vi "addBoolean[]Element.vi"(7 "Name":string, 8 "error in (no error)":errorcluster, 9 "Value":bool[](array[boolean]), 10 "Replace? (false)":bool, 11 "tBSONDocument in":refnum<class "tBSONDocument.lvclass">) -> (0 "error out":errorcluster, 3 "tBSONDocument out":refnum<class "tBSONDocument.lvclass">)   [LabVIEW 2013, in "BSON.lvlib" / "tBSONDocument.lvclass"]
doc: "Adds an array of booleans to a BSON document."
uses:
  tBSONDocument.lvclass
  BSONElements/tBSONBoolean/tBSONBoolean.lvclass
  tBSONElement/tBSONElement.lvclass
  BSONElements/tBSONBoolean/setValue.vi
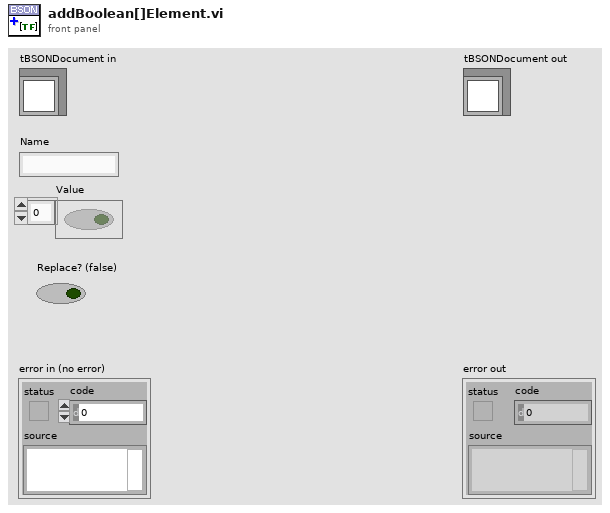
[diagram p1: front panel]
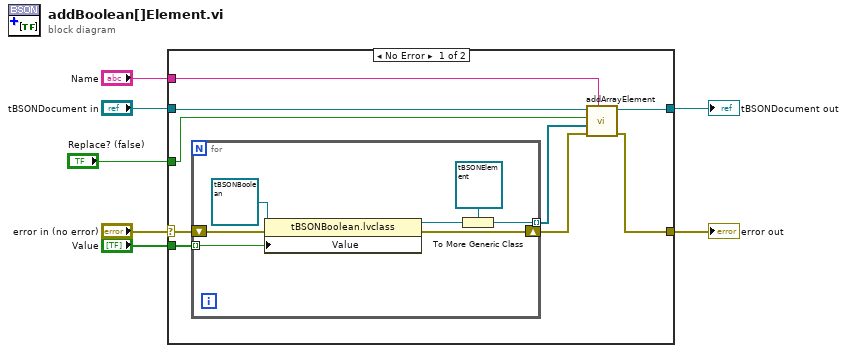
[diagram p0: block diagram]
diagram:
  n1 = case shown="No Error" "error in (no error)" {
    selector: "error in (no error)" -> [w15 w25]
    tunnel: [w10 w25] -> w6
    tunnel: [w9 w24] -> w4
    tunnel: "tBSONDocument in" -> [w14 w24]
    tunnel: "Name" -> [w13 _]
    tunnel: "Value" -> [w16 _]
    tunnel: "Replace? (false)" -> [w8 _]
    frame No Error {
      n2 = for {
        tunnel: w16 -> [w23] mode=indexing
        shift-right: [w20] -> w12
        shift-left: w15 -> [w21]
        tunnel: [w17] -> w11 mode=indexing
        n3 = property class="tBSONBoolean.lvclass"(reference=refnum<class "tBSONBoolean.lvclass"> refnum ("BSON.lvlib:tBSONBoolean.lvclass"), error in=w21, "Value"=w23) -> (reference out=w19:refnum<class "tBSONBoolean.lvclass">, error out=w20:errorcluster)
        n4 = To More Generic Class(target class=refnum<class "tBSONElement.lvclass"> refnum ("BSON.lvlib:tBSONElement.lvclass"), reference=w19) -> (generic class reference=w17:refnum<class "tBSONElement.lvclass">)
      }
      n5 = call "addArrayElement.vi"("Name"=w13, "error in (no error)"=w12, "Value"=w11, "Replace? (false)"=w8, "tBSONDocument in"=w14) -> ("error out"=w10:errorcluster, "tBSONDocument out"=w9:refnum<class "tBSONDocument.lvclass">)  [unwired: 5 in]
    }
    frame Error {
    }
  }
  "error out" <- w6
  "tBSONDocument out" <- w4
